vi "Teleop.vi"(10 "Match Info":T1={"Autonomous Elapsed Seconds"=0.0, "TeleOp Elapsed Seconds"=0.0, "Disabled Elapsed Seconds"=0.0, "Visited Autonomous"=FALSE, "Visited TeleOp"=FALSE, "Visited Disabled"=FALSE, "Autonomous Settings"={"Autonomous Style"=enum."Independent", "VI Refnum"=refnum}}, 11 "Call Context":T2) -> ()   [LabVIEW 2013]
doc: "This VI is called for each TeleOp packet received from the DS where the robot is not disabled. It is often used to read from the joysticks and update I/O or to update setpoints for timed control loops. It should complete and return within 20 milliseconds or it may miss DS packets."
uses:
  <vilib>/Rock Robotics/WPI/DriverStation/WPI_DriverStationDerivedRobotMode.ctl
  <vilib>/Rock Robotics/WPI/DriverStation/WPI_DriverStationMatch Info.ctl
  <vilib>/Rock Robotics/WPI/Solenoid/WPI_SolenoidValue.ctl
  Robot Global Data.vi
  <vilib>/Rock Robotics/WPI/Solenoid/Deprecated/WPI_SolenoidGetBool.vi
  <vilib>/Rock Robotics/WPI/Solenoid/WPI_SolenoidSetEnum.vi
  <vilib>/Rock Robotics/WPI/Joystick/WPI_JoystickGetSetRefNum.vi
  <vilib>/Rock Robotics/WPI/RobotDrive/WPI_RobotDriveGetSetRefNum.vi
panel:
  out "Laser Q2":bool
  out "Laser Q1":bool
  out "Numeric 1":dbl(slide) scale=0.0..100.0
  out "Boolean 2":bool
  out "Boolean 1":bool
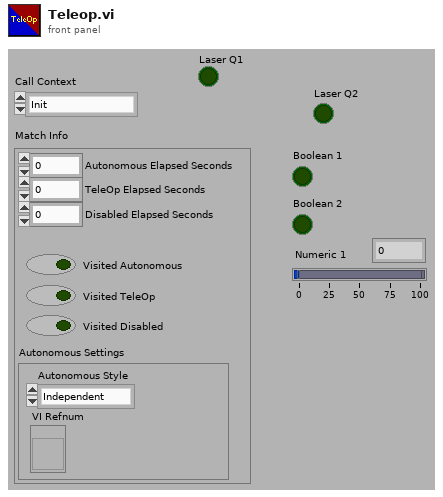
[diagram p1: front panel]
types:
  T1 = typedef "WPI_DriverStationMatch Info.ctl" = cluster{"Autonomous Elapsed Seconds":dbl, "TeleOp Elapsed Seconds":dbl, "Disabled Elapsed Seconds":dbl, "Visited Autonomous":bool, "Visited TeleOp":bool, "Visited Disabled":bool, "Autonomous Settings":cluster{"Autonomous Style":enum16{"Iterative", "Independent"}, "VI Refnum":refnum<vi>}}
  T2 = typedef "WPI_DriverStationDerivedRobotMode.ctl" = enum16{"Init", "Execute", "Stop"}
  T3 = typedef "WPI_DigitalInputDevRef.ctl" = cluster{"DevStatus":errorcluster, "DIO Channel":T4, "Digital Module":T5}
  T4 = typedef "FPGA_DIOChannel.ctl" = enum8{"DIO 1", "DIO 2", "DIO 3", "DIO 4", "DIO 5", "DIO 6", "DIO 7", "DIO 8", "DIO 9", "DIO 10", "DIO 11", "DIO 12", "DIO 13", "DIO 14", "Invalid"}
  T5 = typedef "FPGA_TypedefDigitalModule.ctl" = enum16{"Digital Module 1", "Digital Module 2"}
  T6 = typedef "WPI_RobotDriveDevRef.ctl" = cluster{"DevStatus":errorcluster, "Motors[]":T7[], "Square Inputs":bool, "Max Output":dbl, "Isochronous":bool}
  T7 = typedef "WPI_MotorControlDeviceRef.ctl" = cluster{"DeviceStatus":errorcluster, "Type":enum16{"PWM", "CAN"}, "PWM":cluster{"Digital Module":T5, "PWM Channel":T8, "DeadBand":T9}, "CAN":cluster{"Device Number":u8, "Control Mode":T10, "Semaphore":T11, "Max Vout":dbl}, "Invert":bool, "TransformRef":T12, "InvTransformRef":T12}
  T8 = typedef "FPGA_DIOPWMChannel.ctl" = enum8{"PWM 1", "PWM 2", "PWM 3", "PWM 4", "PWM 5", "PWM 6", "PWM 7", "PWM 8", "PWM 9", "PWM 10", "Invalid"}
  T9 = typedef "WPI_PWMDeadband.ctl" = cluster{"Name":string, "maxPositivePwm":i32, "minPositivePwm":i32, "centerPwm":i32, "maxNegativePwm":i32, "minNegativePwm":i32, "angularRange":u16}
  T10 = typedef "WPI_CANJaguar_ControlMode.ctl" = enum8{"Percent VBus", "Current", "Speed", "Position", "Voltage"}
  T11 = typedef "Semaphore RefNum" = refnum<k1>
  T12 = typedef "WPI_PWMTransform_ConPane.ctl" = refnum<vi>
  T13 = typedef "WPI_JoystickDevRef.ctl" = cluster{"Device":T14}
  T14 = typedef "WPI_JoystickDeviceEnum.ctl" = enum16{"USB 1", "USB 2", "USB 3", "USB 4", "Kinect 1", "Kinect 2"}
  T15 = typedef "WPI_JoystickButtonState.ctl" = cluster{"Button 1":bool, "Button 2":bool, "Button 3":bool, "Button 4":bool, "Button 5":bool, "Button 6":bool, "Button 7":bool, "Button 8":bool, "Button 9":bool, "Button 10":bool, "Button 11":bool, "Button 12":bool}
  T16 = cluster{"axis 1 (x)":dbl, "axis 2 (y)":dbl, "axis 3 (throttle)":dbl, "axis 4":dbl, "axis 5":dbl, "axis 6":dbl}
  T17 = typedef "WPI_AnalogChannelDevRef.ctl" = cluster{"DevStatus":errorcluster, "Analog Module":T18, "Analog Channel":T19}
  T18 = typedef "FPGA_TypedefAnalogModule.ctl" = enum16{"Analog Module 1", "Analog Module 2"}
  T19 = typedef "FPGA_AIChannel.ctl" = enum8{"AI 1", "AI 2", "AI 3", "AI 4", "AI 5", "AI 6", "AI 7", "AI 8", "Invalid"}
  T20 = typedef "WPI_RelayDevRef.ctl" = cluster{"DevStatus":errorcluster, "Relay Channel":T21, "Digital Module":T5, "Relay Direction":T22}
  T21 = typedef "FPGA_DIORelayChannel.ctl" = enum8{"Relay 1", "Relay 2", "Relay 3", "Relay 4", "Relay 5", "Relay 6", "Relay 7", "Relay 8", "Invalid"}
  T22 = typedef "WPI_RelayDirection.ctl" = enum16{"Both directions", "Forward only", "Reverse only"}
  T23 = typedef "WPI_SolenoidValue.ctl" = enum16{"Off", "On", "Forward", "Reverse"}
  T24 = typedef "WPI_SolenoidDevRef.ctl" = cluster{"DevStatus":errorcluster, "Solenoid Module":T25, "Forward Solenoid Channel":T26, "Reverse Solenoid Channel":T26}
  T25 = typedef "FPGA_TypedefSolenoidModule.ctl" = enum16{"Solenoid Module 1", "Solenoid Module 2"}
  T26 = typedef "WPI_SolenoidChannel.ctl" = enum8{"Solenoid 1", "Solenoid 2", "Solenoid 3", "Solenoid 4", "Solenoid 5", "Solenoid 6", "Solenoid 7", "Solenoid 8", "Invalid"}
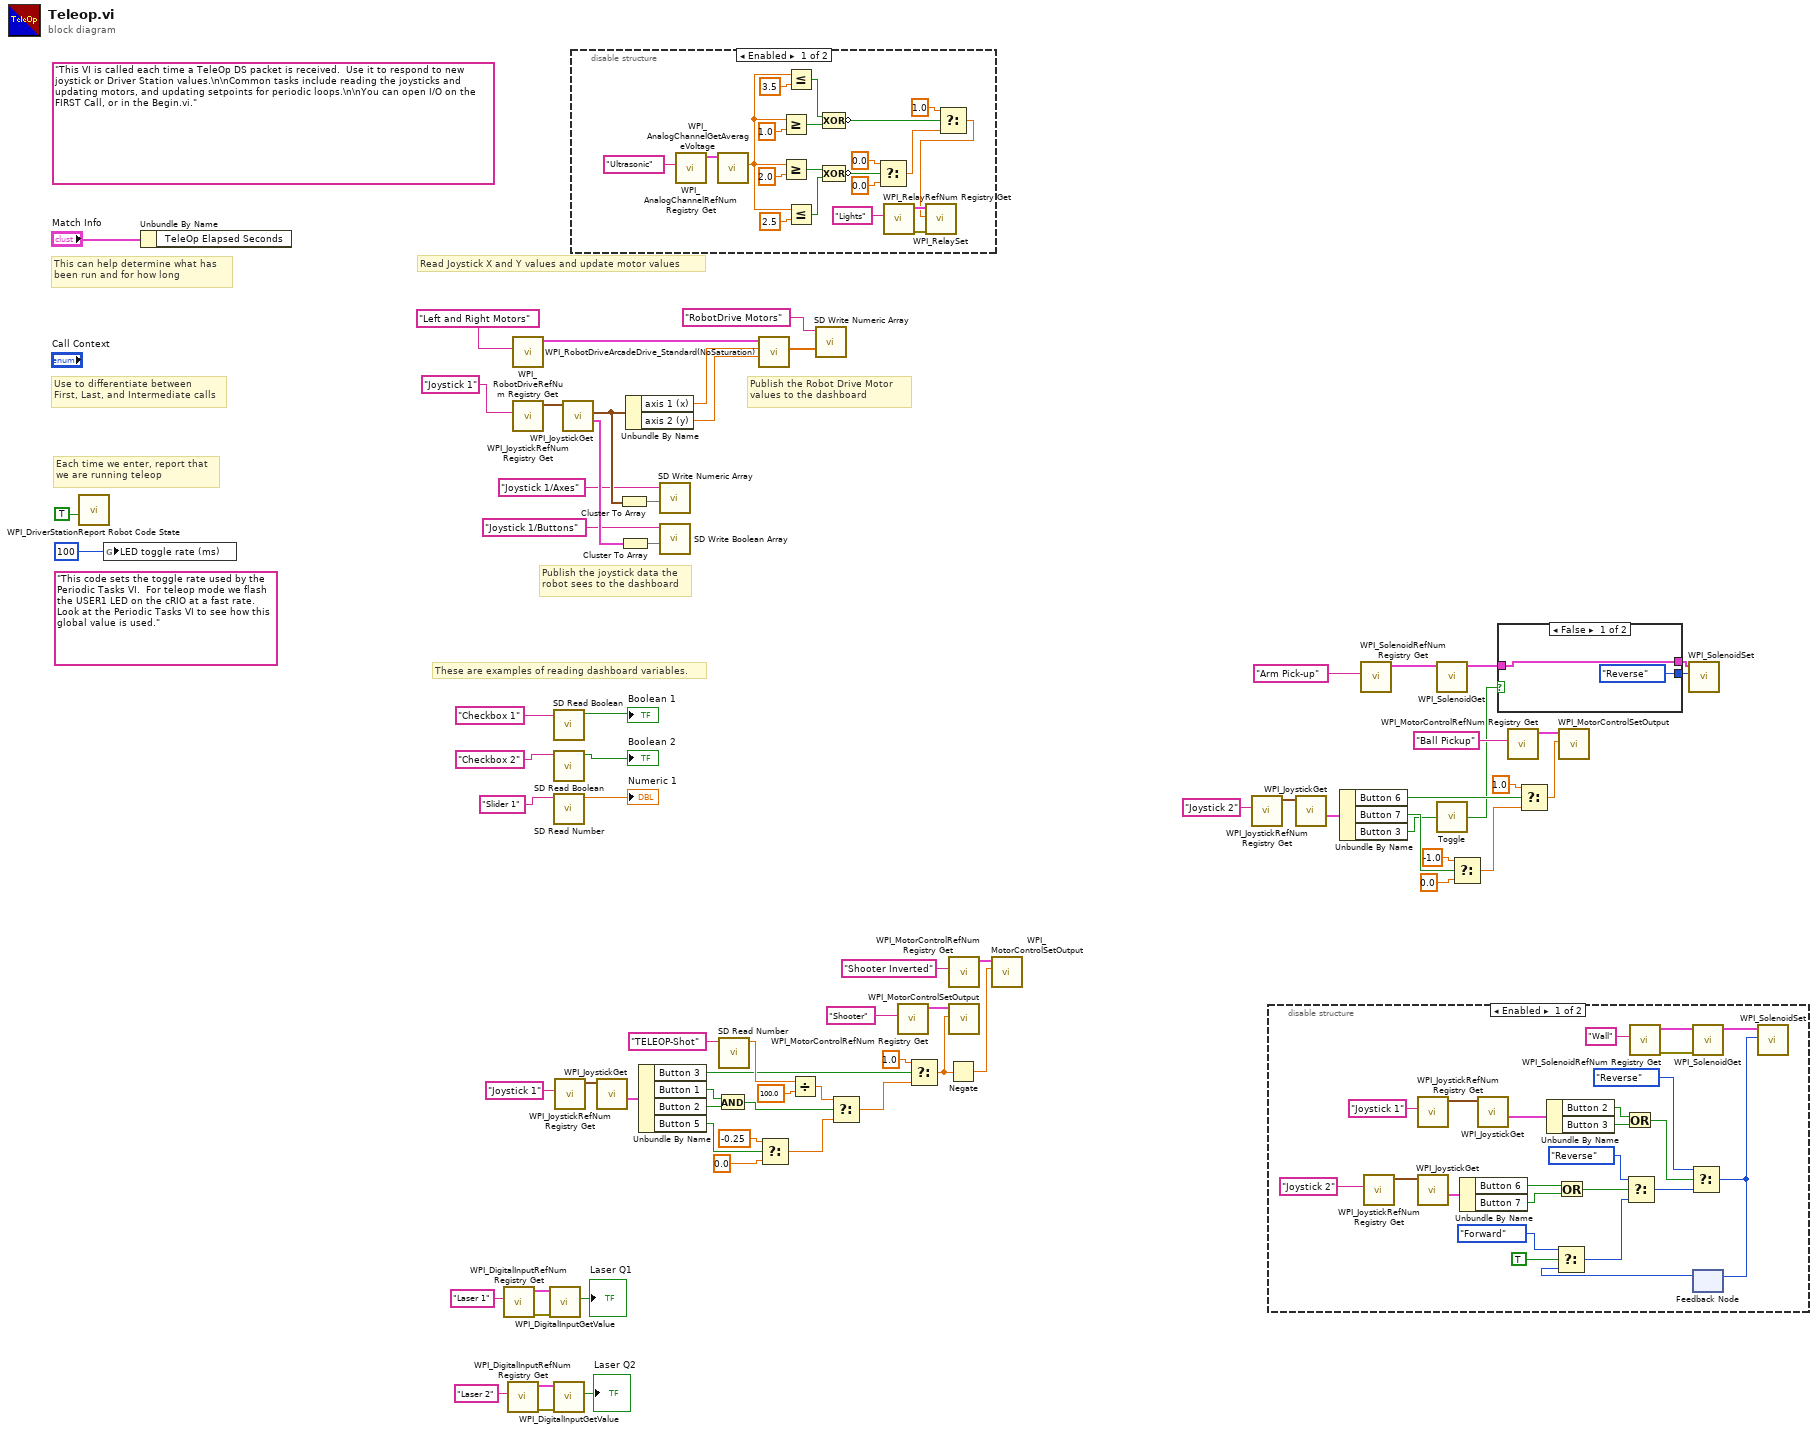
[diagram p0: block diagram]
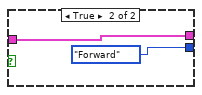
[diagram p4: hidden frame]
diagram:
  (unwired) "This code sets the toggle rate used by the Periodic Tasks VI.  For teleop mode we flash the USER1 LED on the cRIO at a fast rate.  Look at the Periodic Tasks VI to see how this global value is used."
  (unwired) "This VI is called each time a TeleOp DS packet is received.  Use it to respond to new joystick or Driver Station values.\n\nCommon tasks include reading the joysticks and updating motors, and updating setpoints for periodic loops.\n\nYou can open I/O on the FIRST Call, or in the Begin.vi."
  # "These are examples of reading dashboard variables."
  # "Publish the Robot Drive Motor\nvalues to the dashboard"
  # "Publish the joystick data the\nrobot sees to the dashboard"
  # "Each time we enter, report that\nwe are running teleop"
  # "Use to differentiate between\nFirst, Last, and Intermediate calls"
  # "This can help determine what has\nbeen run and for how long"
  # "Read Joystick X and Y values and update motor values"
  n1 = call <vilib>:"WPI_DriverStationReport Robot Code State.vi"("TeleOp"=TRUE ("Autonomous")) -> ()  [unwired: 10 in, 1 out]
  n2 = global write "Robot Global Data.vi" "LED toggle rate (ms)"(u32 100 ("LED ms toggle rate")) -> ()
  n3 = Unbundle By Name("Match Info") -> ()  [unwired: 1 out]
  n4 = call <vilib>:"WPI_DigitalInputRefNum Registry Get.vi"("refnum name"="Laser 1") -> ("error out"=w8:errorcluster, "DigitalInputDevRef"=w7:T3)  [unwired: 9 in]
  n5 = call <vilib>:"WPI_DigitalInputRefNum Registry Get.vi"("refnum name"="Laser 2") -> ("error out"=w1:errorcluster, "DigitalInputDevRef"=w2:T3)  [unwired: 9 in]
  n6 = call <vilib>:"WPI_RobotDriveRefNum Registry Get.vi"("refnum name"="Left and Right Motors") -> ("RobotDriveDevRef"=w71:T6)  [unwired: 1 in, 9 out]
  n7 = call <vilib>:"WPI_JoystickRefNum Registry Get.vi"("refnum name"="Joystick 1") -> ("JoystickDevRef"=w67:T13)  [unwired: 1 in, 9 out]
  n8 = call <vilib>:"WPI_DigitalInputGetValue.vi"("error in (no error)"=w8, "DigitalInputDevRef"=w7) -> ("Value"=→"Laser Q1":bool)  [unwired: 7 in, 2 out]
  n9 = call <vilib>:"SD Read Boolean.vi"("Name"="Checkbox 1" ("refnum name")) -> ("Boolean"=→"Boolean 1":bool)  [unwired: 8 in, 2 out]
  n10 = call <vilib>:"SD Read Boolean.vi"("Name"="Checkbox 2" ("refnum name")) -> ("Boolean"=→"Boolean 2":bool)  [unwired: 8 in, 2 out]
  n11 = call <vilib>:"SD Read Number.vi"("Name"="Slider 1" ("refnum name")) -> ("Numeric"=→"Numeric 1":dbl)  [unwired: 8 in, 2 out]
  n12 = call <vilib>:"WPI_DigitalInputGetValue.vi"("error in (no error)"=w1, "DigitalInputDevRef"=w2) -> ("Value"=→"Laser Q2":bool)  [unwired: 7 in, 2 out]
  n13 = call <vilib>:"WPI_JoystickRefNum Registry Get.vi"("refnum name"="Joystick 1") -> ("JoystickDevRef"=w49:T13)  [unwired: 1 in, 9 out]
  n14 = call <vilib>:"WPI_JoystickGet.vi"("JoystickDevRef"=w67) -> ("Buttons"=w64:T15, "Axes"=w61:T16)  [unwired: 1 in, 4 out]
  n15 = disable-structure shown="Enabled" {
    frame Enabled {
      n16 = call <vilib>:"WPI_AnalogChannelRefNum Registry Get.vi"("refnum name"="Ultrasonic") -> ("AIDeviceRef"=w93:T17)  [unwired: 9 in, 1 out]
      n17 = call <vilib>:"WPI_AnalogChannelGetAverageVoltage.vi"("AIDeviceRef"=w93) -> ("Voltage"=w84:dbl)  [unwired: 8 in, 2 out]
      n18 = Greater Or Equal?(x=w84, y=1.0) -> (x >= y?=w87:bool)
      n19 = Greater Or Equal?(x=w84, y=2.0) -> (x >= y?=w81:bool)
      n20 = Less Or Equal?(x=w84, y=3.5) -> (x <= y?=w86:bool)
      n21 = Less Or Equal?(x=w84, y=2.5) -> (x <= y?=w82:bool)
      n22 = Compound Arithmetic op=XOR(w86, w87) -> (invert w79:bool)
      n23 = Compound Arithmetic op=XOR(w81, w82) -> (invert w80:bool)
      n24 = Select(t=0.0, s=w80, f=0.0) -> (s? t:f=w75:dbl)
      n25 = call <vilib>:"WPI_RelayRefNum Registry Get.vi"("refnum name"="Lights") -> ("error out"=w92:errorcluster, "RelayDevRef"=w91:T20)  [unwired: 9 in]
      n26 = Select(t=1.0, s=w79, f=w75) -> (s? t:f=w74:dbl)
      n27 = call <vilib>:"WPI_RelaySet.vi"("error in (no error)"=w92, "RelayValue"=w74, "RelayDevRef"=w91) -> ()  [unwired: 7 in, 2 out]
    }
    frame Disabled {
    }
  }
  n28 = call <vilib>:"WPI_JoystickGet.vi"("JoystickDevRef"=w49) -> ("Buttons"=w48:T15)  [unwired: 1 in, 5 out]
  n29 = Cluster To Array(cluster=w61) -> (array=w60:dbl[])
  n30 = Cluster To Array(cluster=w64) -> (array=w63:bool[])
  n31 = Unbundle By Name(w61) -> ("axis 1 (x)"=w70:dbl, "axis 2 (y)"=w69:dbl)
  n32 = Unbundle By Name(w48) -> ("Button 3"=w12:bool, "Button 1"=w17:bool, "Button 2"=w18:bool, "Button 5"=w46:bool)
  n33 = call <vilib>:"SD Write Numeric Array.vi"("Numeric Array"=w60, "Name"="Joystick 1/Axes") -> ()  [unwired: 8 in, 2 out]
  n34 = call <vilib>:"SD Write Boolean Array.vi"("Boolean Array"=w63, "Name"="Joystick 1/Buttons") -> ()  [unwired: 8 in, 2 out]
  n35 = And(x=w17, y=w18) -> (x .and. y?=w47:bool)
  n36 = call <vilib>:"SD Read Number.vi"("Name"="TELEOP-Shot") -> ("Numeric"=w15:dbl)  [unwired: 8 in, 2 out]
  n37 = call <vilib>:"WPI_RobotDriveArcadeDrive_Standard(NoSaturation).vi"("Y axis value"=w69, "X axis value"=w70, "RobotDriveDevRef"=w71) -> ("Motor Values"=w57:dbl[])  [unwired: 1 in, 7 out]
  n38 = Select(t=-0.25, s=w46, f=0.0) -> (s? t:f=w43:dbl)
  n39 = Divide(x=w15, y=100.0) -> (x/y=w13:dbl)
  n40 = call <vilib>:"SD Write Numeric Array.vi"("Numeric Array"=w57, "Name"="RobotDrive Motors") -> ()  [unwired: 8 in, 2 out]
  n41 = Select(t=w13, s=w47, f=w43) -> (s? t:f=w11:dbl)
  n42 = call <vilib>:"WPI_MotorControlRefNum Registry Get.vi"("refnum name"="Shooter") -> ("MotorControlDevRef"=w41:T7)  [unwired: 9 in, 1 out]
  n43 = Select(t=1.0, s=w12, f=w11) -> (s? t:f=w9:dbl)
  n44 = Negate(x=w9) -> (-x=w39:dbl)
  n45 = call <vilib>:"WPI_MotorControlRefNum Registry Get.vi"("refnum name"="Shooter Inverted") -> ("MotorControlDevRef"=w38:T7)  [unwired: 9 in, 1 out]
  n46 = call <vilib>:"WPI_MotorControlSetOutput.vi"("Output"=w9, "MotorControlDevRef"=w41) -> ()  [unwired: 7 in, 3 out]
  n47 = call <vilib>:"WPI_MotorControlSetOutput.vi"("Output"=w39, "MotorControlDevRef"=w38) -> ()  [unwired: 7 in, 3 out]
  n48 = call <vilib>:"WPI_JoystickRefNum Registry Get.vi"("refnum name"="Joystick 2") -> ("JoystickDevRef"=w37:T13)  [unwired: 1 in, 9 out]
  n49 = disable-structure shown="Enabled" {
    frame Enabled {
      n50 = call <vilib>:"WPI_JoystickRefNum Registry Get.vi"("refnum name"="Joystick 2") -> ("JoystickDevRef"=w118:T13)  [unwired: 9 in, 1 out]
      n51 = call <vilib>:"WPI_JoystickRefNum Registry Get.vi"("refnum name"="Joystick 1") -> ("JoystickDevRef"=w117:T13)  [unwired: 9 in, 1 out]
      n52 = call <vilib>:"WPI_JoystickGet.vi"("JoystickDevRef"=w118) -> ("Buttons"=w113:T15)  [unwired: 4 in, 2 out]
      n53 = Unbundle By Name(w113) -> ("Button 6"=w100:bool, "Button 7"=w99:bool)
      n54 = call <vilib>:"WPI_JoystickGet.vi"("JoystickDevRef"=w117) -> ("Buttons"=w114:T15)  [unwired: 4 in, 2 out]
      n55 = Unbundle By Name(w114) -> ("Button 2"=w97:bool, "Button 3"=w96:bool)
      n56 = Or(x=w100, y=w99) -> (x .or. y?=w98:bool)
      n57 = Or(x=w97, y=w96) -> (x .or. y?=w95:bool)
      n58 = call <vilib>:"WPI_SolenoidRefNum Registry Get.vi"("refnum name"="Wall") -> ("error out"=w104:errorcluster, "SolenoidDevRef"=w105:T24)  [unwired: 9 in]
      n59 = call-poly <vilib>:"WPI_SolenoidGet.vi"("error in (no error)"=w104, "SolenoidDevRef"=w105) -> ("SolenoidDevRef"=w103:T24)  [unwired: 7 in, 2 out]
      n60 = feedback #1() -> (w101:T23)  [unwired: 1 in]
      n61 = Select(t=WPI_SolenoidValue."Forward" ("Value"), s=TRUE, f=w101) -> (s? t:f=w108:T23)
      n62 = Select(t=WPI_SolenoidValue."Reverse" ("Value"), s=w98, f=w108) -> (s? t:f=w107:T23)
      n63 = Select(t=WPI_SolenoidValue."Reverse" ("Value"), s=w95, f=w107) -> (s? t:f=w102:T23)
      n64 = feedback-in #1(w102) -> ()
      n65 = call-poly <vilib>:"WPI_SolenoidSet.vi"("Value"=w102, "SolenoidDevRef"=w103) -> ()  [unwired: 8 in, 2 out]
    }
    frame Disabled {
    }
  }
  n66 = call <vilib>:"WPI_JoystickGet.vi"("JoystickDevRef"=w37) -> ("Buttons"=w35:T15)  [unwired: 1 in, 5 out]
  n67 = Unbundle By Name(w35) -> ("Button 6"=w33:bool, "Button 7"=w34:bool, "Button 3"=w25:bool)
  n68 = call <vilib>:"WPI_SolenoidRefNum Registry Get.vi"("refnum name"="Arm Pick-up") -> ("SolenoidDevRef"=w23:T24)  [unwired: 9 in, 1 out]
  n69 = call-poly <vilib>:"WPI_SolenoidGet.vi"("SolenoidDevRef"=w23) -> ("SolenoidDevRef"=w22:T24)  [unwired: 8 in, 2 out]
  n70 = call "Toggle.vi"("Input"=w25) -> ("Toggled Output"=w24:bool)
  n71 = Select(t=-1.0, s=w34, f=0.0) -> (s? t:f=w29:dbl)
  n72 = case shown="False" w24 {
    tunnel: w22 -> [w120 w122]
    tunnel: [w120 w122] -> w20
    tunnel: [WPI_SolenoidValue."Reverse" ("Value") WPI_SolenoidValue."Forward" ("Value")] -> w19
    frame False {
    }
    frame True {
    }
  }
  n73 = call <vilib>:"WPI_MotorControlRefNum Registry Get.vi"("refnum name"="Ball Pickup") -> ("MotorControlDevRef"=w27:T7)  [unwired: 9 in, 1 out]
  n74 = Select(t=1.0, s=w33, f=w29) -> (s? t:f=w26:dbl)
  n75 = call <vilib>:"WPI_MotorControlSetOutput.vi"("Output"=w26, "MotorControlDevRef"=w27) -> ()  [unwired: 7 in, 3 out]
  n76 = call-poly <vilib>:"WPI_SolenoidSet.vi"("Value"=w19, "SolenoidDevRef"=w20) -> ()  [unwired: 8 in, 2 out]
